vi "fgt set sensor Regulation.vi"(8 "error in (no error)":errorcluster, 9 "setpoint":sgl, 10 "pressureIndex":u32, 11 "sensorIndex":u32) -> (0 "error out":errorcluster)   [LabVIEW 2016, in "fgt_SDK.lvlib"]
doc: "Start closed loop regulation between a sensor and a pressure controller. Pressure will be regulated in order to reach sensor setpoint.\nCall again this function in order to change the setpoint. Calling fgt_set_pressure on same pressureIndex will stop regulation."
uses:
  fgt_SDK.lvlib
  dlls/fgt_SDK_32.dll
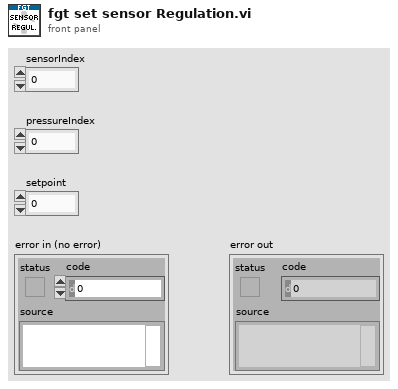
[diagram p1: front panel]
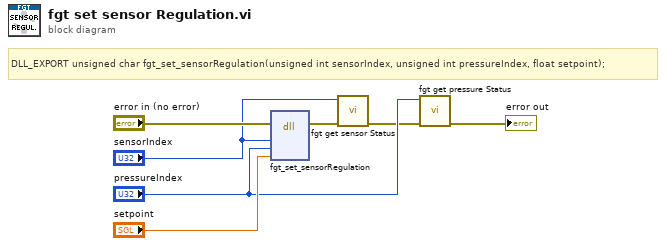
[diagram p0: block diagram]
diagram:
  # "DLL_EXPORT unsigned char fgt_set_sensorRegulation(unsigned int sensorIndex, unsigned int pressureIndex, float setpoint);"
  n1 = dll-call lib="PTH2Zabs D\nMes DocumentsDéveloppementFluigentSDKsfgt-sdk-labviewdllsfgt_SDK_*.*" fn="fgt_set_sensorRegulation"(error in="error in (no error)", "sensorIndex"="sensorIndex", "pressureIndex"="pressureIndex", "setpoint"="setpoint") -> (error out=w5:errorcluster)  [unwired: 6 in, 1 out]
  n2 = call "fgt get sensor Status.vi"("error in (no error)"=w5, "pressureIndex"="sensorIndex") -> ("error out"=w2:errorcluster)  [unwired: 9 in]
  n3 = call "fgt get pressure Status.vi"("error in (no error)"=w2, "pressureIndex"="pressureIndex") -> ("error out"=→"error out":errorcluster)  [unwired: 9 in]
